vi "DC Voltage.vi"() -> ()   [LabVIEW 2021]
uses:
  <vilib>/LabVIEW Interface for Arduino/LabVIEW Interface for Arduino.lvlib
panel:
  out "error out":errorcluster
  in  "stop":bool
  in  "VISA resource":refnum<visa-resource-name>
  out "Voltage":dbl(knob) scale=0.0..5.0
  in  "Analog Input Pin (0)":u8
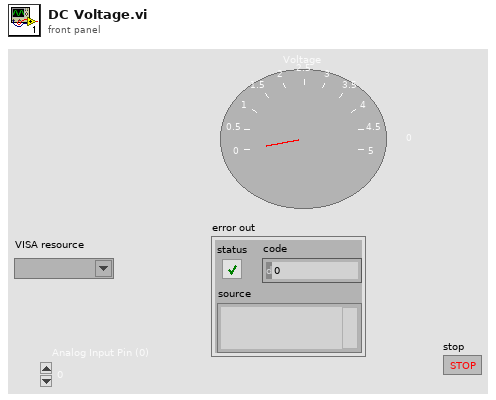
[diagram p1: front panel]
types:
  T1 = typedef "LabVIEW Interface for Arduino.lvlib/Arduino Resource.ctl" = cluster{"VISA resource":refnum<visa-resource-name>, "Board Type":T2, "Connection Type":enum8{"USB / Serial"}, "Bytes Per Packet (15)":u8}
  T2 = typedef "LabVIEW Interface for Arduino.lvlib/Board Type.ctl" = enum16{"Uno", "Dimuelanove w/Atmega 328", "Mega 2560"}
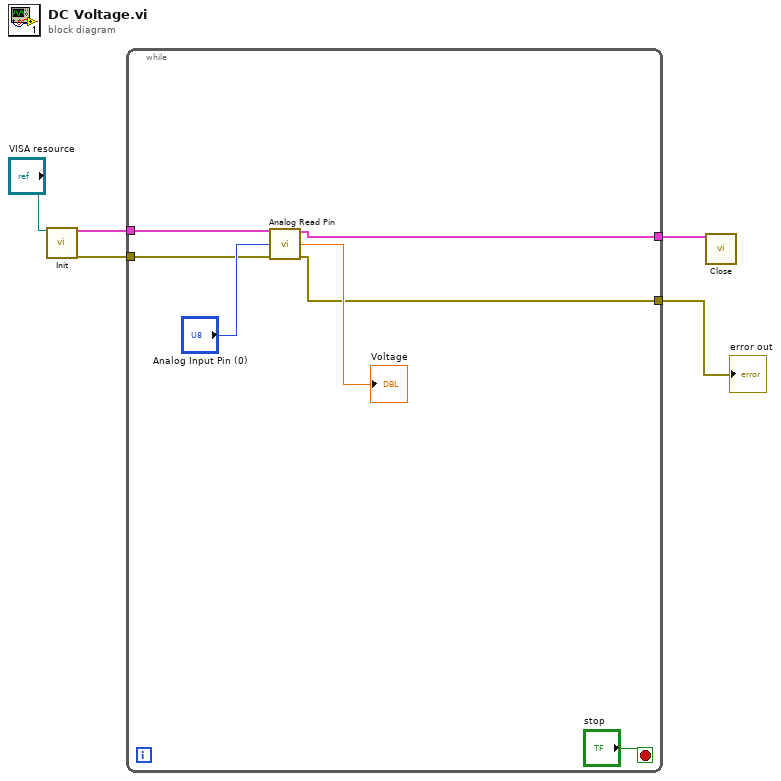
[diagram p0: block diagram]
diagram:
  n1 = call <vilib>:"Init.vi"("VISA resource"="VISA resource") -> ("Arduino Resource"=w5:T1, "error out"=w3:errorcluster)  [unwired: 17 in]
  n2 = while {
    tunnel: w5 -> [w12]
    tunnel: [w11] -> w4
    tunnel: w3 -> [w9]
    tunnel: [w6] -> w1
    stop <- "stop" stop-if-true
    n3 = call <vilib>:"Analog Read Pin.vi"("Arduino Resource"=w12, "Analog Input Pin (0)"="Analog Input Pin (0)", "error in"=w9) -> ("Arduino Resource"=w11:T1, "Voltage"=→"Voltage":dbl, "error out"=w6:errorcluster)  [unwired: 10 in]
  }
  "error out" <- w1
  n4 = call <vilib>:"Close.vi"("Arduino Resource"=w4) -> ()  [unwired: 14 in, 1 out]
